vi "AnalyzePointing.vi"() -> ()   [LabVIEW 2011]
panel:
  in  "file name":string
  in  "folder":path
  in  "Info":string
  out "Plot Images:Front 2":picture
  out "standard deviation total":dbl format="%0.2f"
  out "standard deviation 2":dbl format="%0.2f"
  out "standard deviation":dbl format="%0.2f"
  out "Waveform Graph":dbl[][](graph)
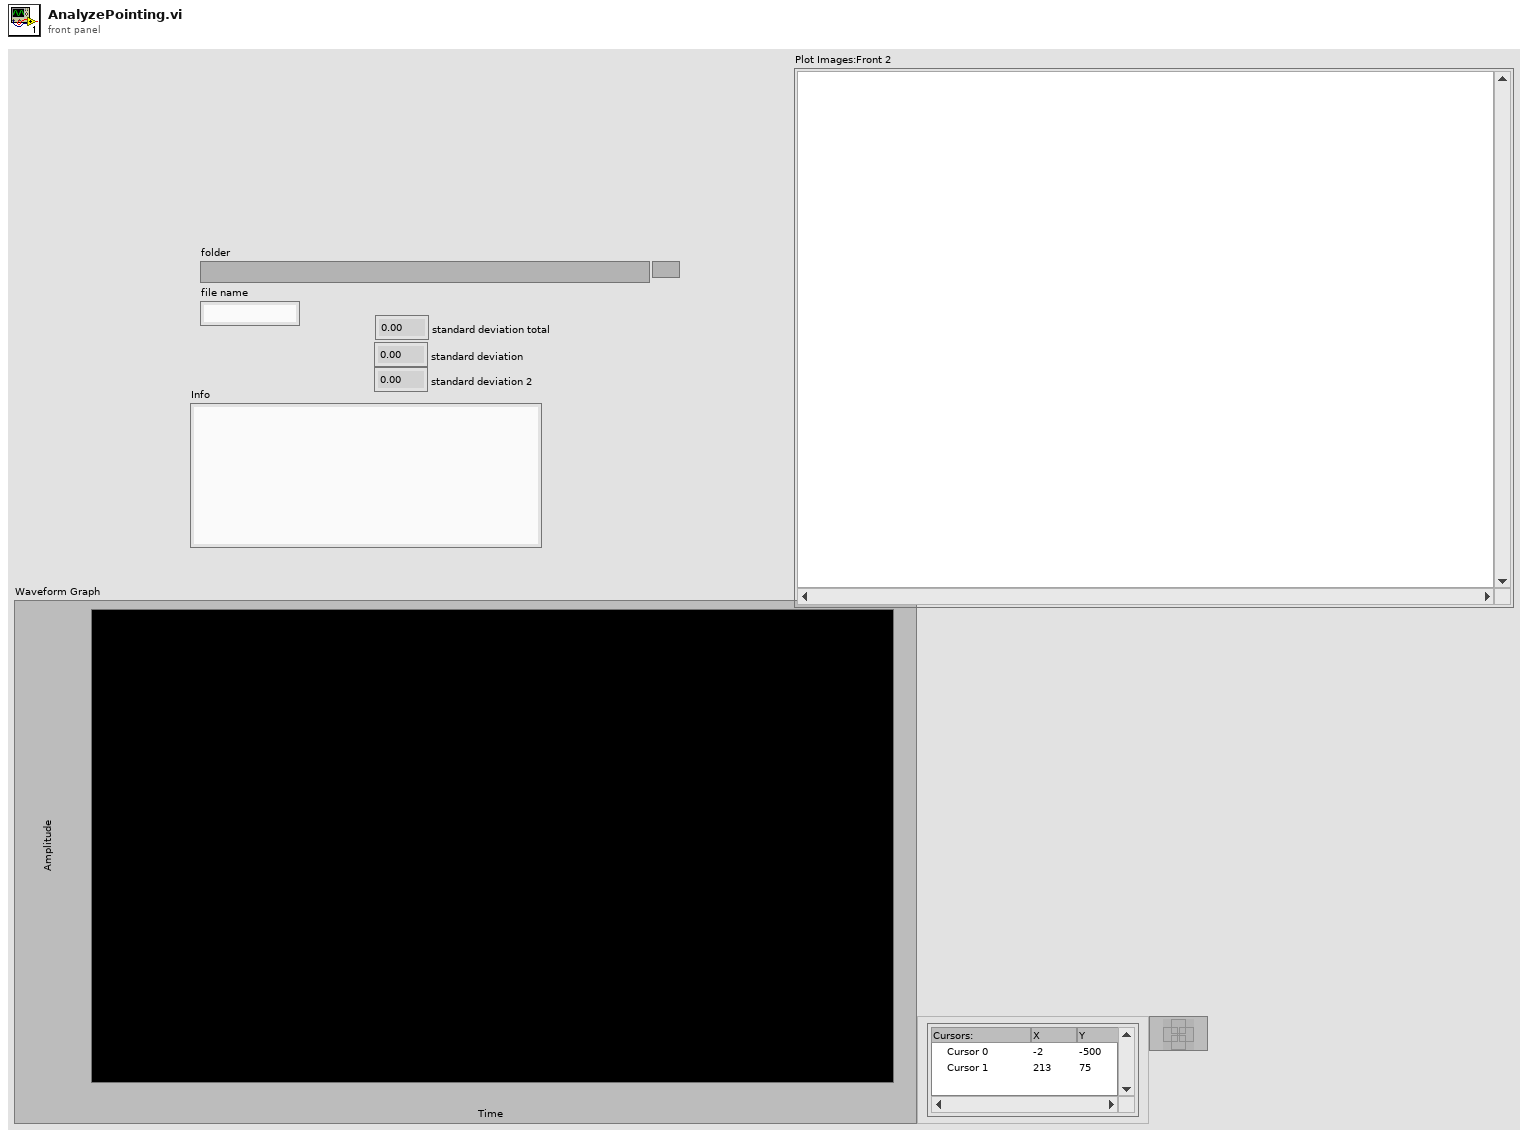
[diagram p1: front panel]
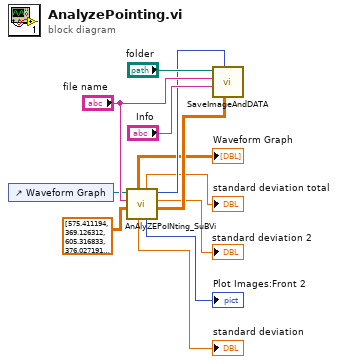
[diagram p0: block diagram]
diagram:
  n1 = control-ref of="Waveform Graph"() -> (w7:refnum<vi>)
  n2 = call "AnAlyZEPoINting_SuBVi.vi"("Array in"=dbl[][] [[575.411194, 369.126312], [605.316833, 376.027191], [579.988159, 388.125488], [580.378845, 349.661224], [585.863892, 388.480713], [584.661865, 368.671783], [553.878357, 366.099335], [581.317017, 344.510437], [574.280884, 352.145538], [556.785522, 366.304474], [585.602417, 378.279449], [594.53302, 357.299896], [564.910767, 355.487305], [566.309265, 364.928284], [570.624695, 334.778564], [570.883301, 358.229492], [576.530701, 370.069885], [574.610596, 378.615814], [571.908752, 353.16275], [585.766052, 365.97876], [557.185852, 356.868591], [554.424194, 378.185547], [546.981018, 370.11792], [568.902771, 381.656342], [563.787476, 390.445679], [552.395203, 385.911743], [570.10199, 353.804291], [583.559448, 368.970795], [613.877747, 373.99408], [554.592407, 383.134796], [590.197815, 395.213318], [563.496765, 380.507019], [568.165771, 398.266235], [554.349121, 395.36377], [577.035889, 398.334412], [570.022583, 395.139648], [556.327026, 401.844025], [594.665405, 385.828827], [565.340759, 343.620117], [577.920898, 376.238861], [573.008545, 374.387451], [580.620972, 412.417297], [570.498169, 376.098969], [568.052673, 346.049286], [579.220093, 380.759705], [583.569824, 379.512878], [579.53064, 381.28595], [557.109253, 364.359985], [589.828125, 395.083557], [573.022583, 367.061066], [587.579224, 378.346436], [573.360657, 369.821625], [589.310974, 363.570587], [568.935913, 365.189392], [587.040466, 377.113983], [556.540771, 349.185944], [581.78241, 380.417297], [579.838684, 360.295837], [558.146301, 371.600342], [548.877136, 353.046051], [577.533691, 377.653931], [558.154053, 364.863922], [539.90863, 359.460083], [576.077515, 342.370636], [559.963623, 374.365723], [555.805542, 365.507294], [580.674805, 373.586823], [579.169617, 369.076538], [574.947632, 359.055542], [569.174683, 371.383881], [563.254761, 360.522919], [588.752869, 348.431793], [564.992249, 369.623932], [569.673279, 370.521393], [564.858459, 371.016266], [554.608215, 343.030121], [565.545105, 359.560211], [585.675964, 366.034668], [573.312195, 355.73465], [556.470032, 361.118195], [571.2276, 378.264557], [570.703125, 332.652771], [570.082397, 362.914032], [566.761658, 349.344635], [572.478516, 364.258301], [576.248657, 349.44101], [571.909302, 347.006714], [571.490112, 384.21048], [571.617004, 356.110687], [559.62262, 352.315704], [583.723938, 360.698425], [566.416809, 379.424408], [582.956299, 371.977722], [583.37146, 331.073822], [579.17627, 396.455414], [570.326172, 366.075073], [561.880981, 331.524689], [559.171753, 347.531006], [580.142578, 346.088348], [570.176575, 354.917145], [582.441589, 380.136658], [578.335999, 374.346558], [593.278198, 369.405548], [564.527588, 348.143677], [579.655396, 375.138275], [577.049927, 371.800232], [580.093689, 354.830322], [554.409302, 379.669708], [559.599426, 390.045013], [575.057495, 373.234528], [585.736206, 365.242737], [590.52832, 375.822418], [580.579956, 375.714172], [576.052856, 358.922272], [558.045532, 349.19455], [564.973511, 342.179535], [579.452942, 381.424103], [558.22583, 353.15506], [593.082947, 358.063538], [568.881287, 349.726105], [580.458618, 360.047546], [597.811462, 346.487701], [573.610718, 361.64505], [550.46228, 359.893829], [585.101379, 353.940094], [567.885132, 366.80191], [566.145996, 367.885895], [561.748291, 373.126953], [551.36322, 369.821869], [546.8302, 363.730225], [578.309326, 354.404449], [598.694885, 372.945312], [569.794983, 364.779938], [566.846436, 320.579437], [573.196533, 342.426788], [588.776245, 370.010925], [566.00769, 367.572235], [570.555969, 396.637207], [572.117065, 389.143494], [556.196655, 396.176758], [572.349487, 366.497131], [579.537598, 386.502747], [567.3255, 397.817993], [578.13562, 379.374268], [571.216492, 397.842834], [570.679993, 388.551392], [567.115051, 372.560822], [565.935791, 376.963074], [577.272156, 372.886993], [555.67688, 384.506104], [582.987671, 378.549988], [582.339539, 361.977142], [570.814209, 377.562164], [560.209229, 381.947876], [578.422119, 402.210571], [584.379822, 372.016205], [569.936035, 372.670685], [571.63446, 366.655609], [543.762329, 381.113647], [562.911316, 365.345367], [563.691956, 368.714417], [573.417297, 371.755096], [569.75238, 364.392761], [574.708069, 364.582306], [569.895325, 385.954773], [566.234863, 381.995453], [582.537537, 366.495331], [566.343689, 361.662201], [575.510071, 339.647034], [576.924805, 352.590668], [572.807495, 379.447449], [582.815125, 337.675964], [562.774475, 372.548737], [572.810852, 379.352875], [552.767578, 369.162994], [568.832458, 354.458588], [575.572876, 377.790497], [558.378784, 357.011597], [554.462036, 378.603363], [552.707825, 358.106262], [572.73938, 346.691467], [551.941833, 318.678741], [549.018494, 330.195618], [583.763489, 357.583282], [582.698792, 359.463196], [568.702576, 364.897522], [563.194031, 337.47052], [561.799988, 357.012329], [576.766113, 356.953461], [572.296448, 351.158691], [567.432373, 345.037903], [540.953918, 353.672119], [573.146362, 325.218994], [564.212952, 349.101501], [558.07666, 345.612091], [567.21521, 339.014679], [574.486328, 393.578064], [577.806213, 285.717743], [585.369446, 371.750397], [586.878113, 359.982697], [561.945862, 341.22052], [572.42157, 364.450073], [560.891785, 344.344391], [562.043091, 344.755493], [580.385437, 351.367523], [580.299927, 350.933563], [548.618347, 352.456238], [570.151672, 341.577454], [572.567505, 370.35437], [571.668823, 369.384308], [570.023071, 348.460724], [553.521179, 360.835937], [560.58252, 339.082581], [572.297791, 361.69516]] ("Array"), "file name"="file name", "WaveformGraph in"=w7) -> ("Array out"=w12:dbl[][], "standard deviation 2"=→"standard deviation 2":dbl, "new picture"=w8:picture, "Plot Images:Front 2"=→"Plot Images:Front 2":picture, "standard deviation total"=→"standard deviation total":dbl, "standard deviation"=→"standard deviation":dbl, "Waveform Graph"=→"Waveform Graph":dbl[][])  [unwired: 2 in]
  n3 = call "SaveImageAndDATA.vi"("Array"=w12, "new picture"=w8, "Info"="Info", "file name"="file name", "folder"="folder") -> ()  [unwired: 7 in]
